vi "Check_if_activated (SubVI).vi"(7 "Override":bool, 9 "activate  every  iterations":i32, 10 "activated?":bool, 11 "Iteration":i32) -> (3 "perform action":bool)   [LabVIEW 2014]
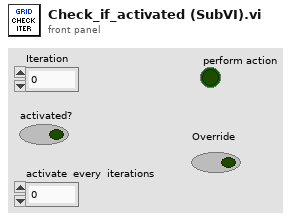
[diagram p1: front panel]
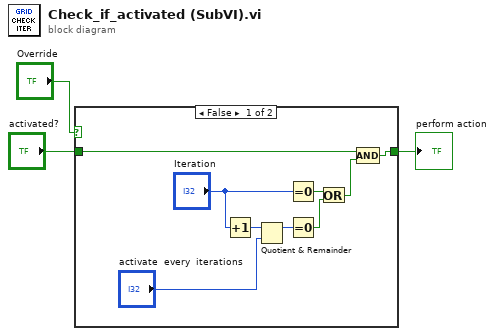
[diagram p0: block diagram]
diagram:
  n1 = case shown="False" "Override" {
    tunnel: "activated?" -> [w7 w13]
    tunnel: [w9 w13] -> w2
    frame False {
      n2 = Increment(x="Iteration") -> (x+1=w11:i32)
      n3 = Quotient & Remainder(x=w11, y="activate  every  iterations") -> (x-y*floor(x/y)=w10:i32)  [unwired: 1 out]
      n4 = Equal To 0?(x="Iteration") -> (x = 0?=w4:bool)
      n5 = Equal To 0?(x=w10) -> (x = 0?=w8:bool)
      n6 = Or(x=w4, y=w8) -> (x .or. y?=w5:bool)
      n7 = Compound Arithmetic op=AND(w7, w5) -> (w9:bool)
    }
    frame True {
    }
  }
  "perform action" <- w2
